vi "CompareMaxMin.vi"(1 "Min":dbl format="%#_10f", 2 "X":dbl format="%#_10f", 3 "Max":dbl format="%#_10f") -> (0 "OutCompare":bool)   [LabVIEW 2018]
panel:
  out "x <= y?":bool
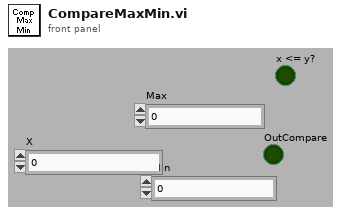
[diagram p1: front panel]
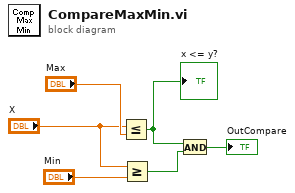
[diagram p0: block diagram]
diagram:
  n1 = Less Or Equal?(x="X", y="Max") -> (x <= y?=w3:bool)
  "x <= y?" <- w3
  n2 = Greater Or Equal?(x="X", y="Min") -> (x >= y?=w2:bool)
  n3 = And(x=w3, y=w2) -> (x .and. y?=→"OutCompare":bool)
